vi "SUB_TextRunList_Color.vi"(3 "Current Step":i32, 4 "Totally Test Items":i32, 5 "List run file":string[](array[string])) -> (1 "ListFile":cluster{"Result":bool, string}[](array[cluster]))   [LabVIEW 2011]
panel:
  out "exeFilename":string
  in  "Result":bool
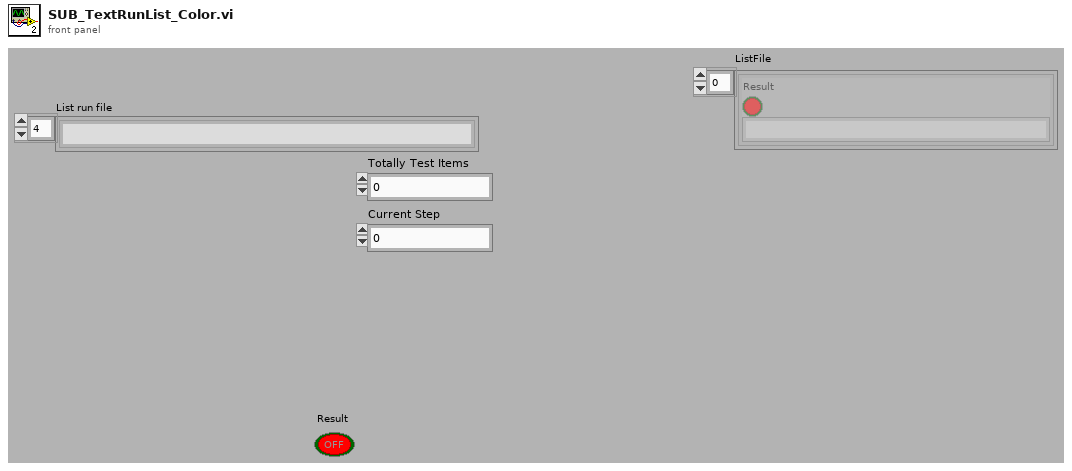
[diagram p1: front panel]
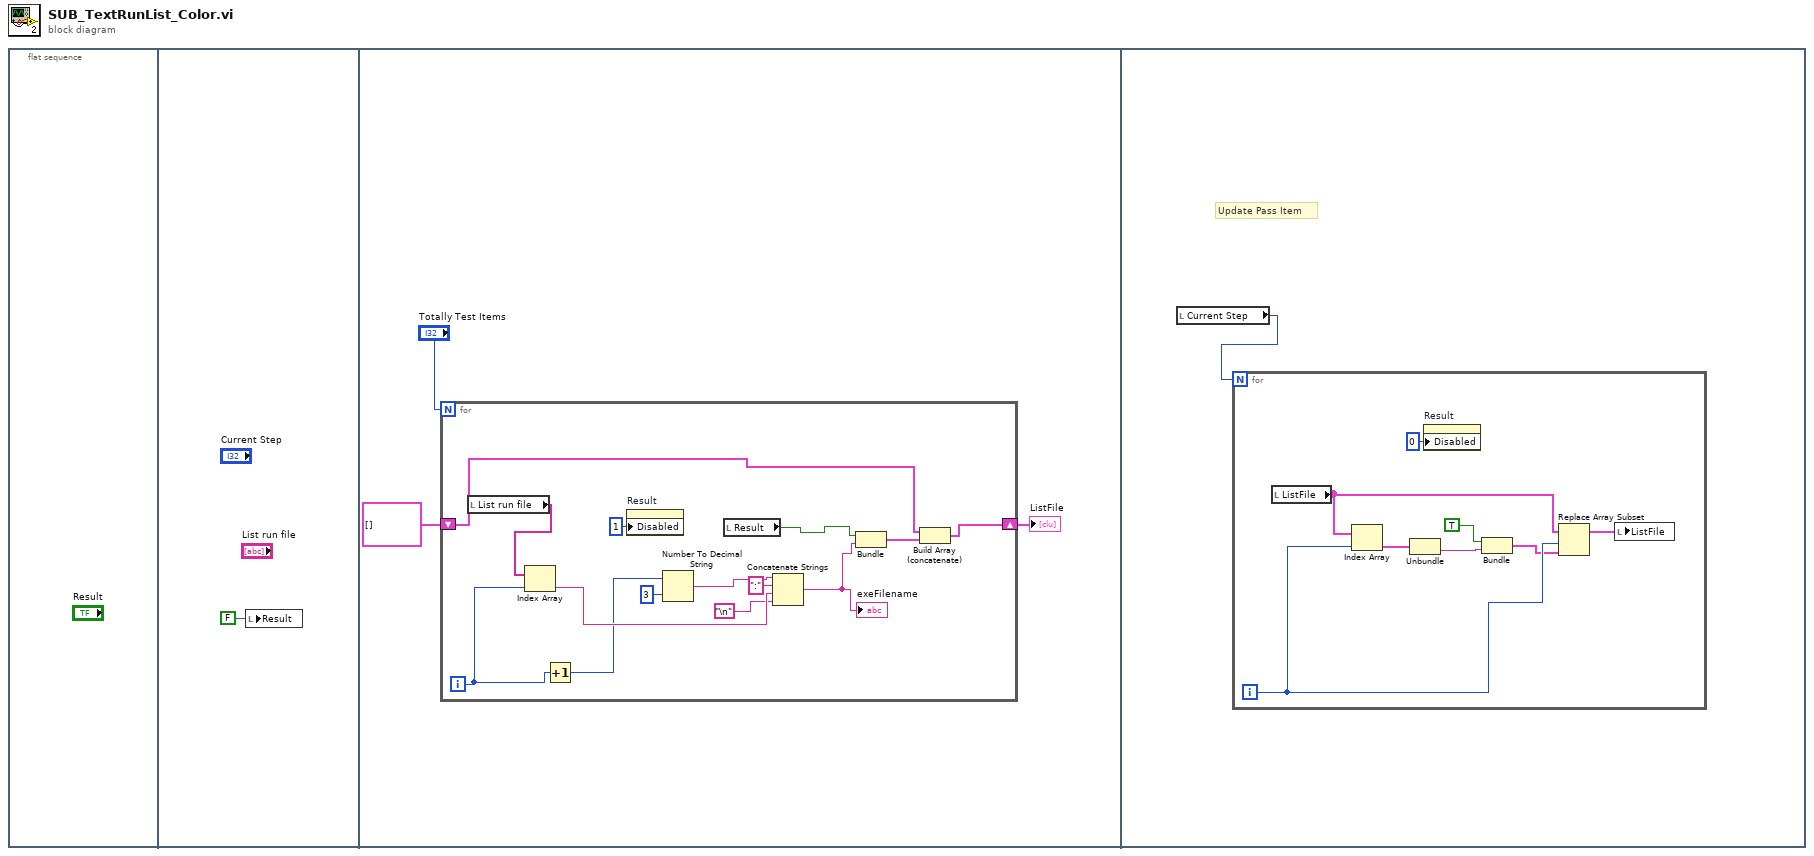
[diagram p0: block diagram]
diagram:
  n1 = flat-sequence {
    frame #0 {
    }
    frame #1 {
      n2 = local write "Result"(FALSE ("Result")) -> ()
    }
    frame #2 {
      n3 = for {
        N: "Totally Test Items" -> [_]
        shift-right: [w12] -> w3
        shift-left: cluster{"Result":bool, string}[] [] -> [w11]
        i -> [w8]
        n4 = local read "List run file"() -> (w18:string[])
        n5 = Index Array(array=w18, index=w8) -> (element=w14:string)
        n6 = Increment(x=w8) -> (x+1=w7:i32)
        n7 = property on="Result" class="Bool (strict)"("Disabled"=u8 1) -> ()  [unwired: 2 in, 2 out]
        n8 = Number To Decimal String(number=w7, width (-)=i16 3) -> (decimal integer string=w16:string)
        n9 = local read "Result"() -> (w6:bool)
        n10 = Concatenate Strings(w16, ":" ("string"), w14, "\n") -> (w10:string)
        "exeFilename" <- w10
        n11 = Bundle("Result"=w6, w10) -> (w9:cluster{"Result":bool, string})  [unwired: 1 in]
        n12 = Build Array (concatenate)(w11, w9) -> (w12:cluster{"Result":bool, string}[])
      }
      "ListFile" <- w3
    }
    frame #3 {
      # "Update Pass Item"
      n13 = local read "Current Step"() -> (w19:i32)
      n14 = for {
        N: w19 -> [_]
        i -> [w23]
        n15 = local read "ListFile"() -> (w24:cluster{"Result":bool, string}[])
        n16 = Index Array "Index Array"(array=w24, index=w23) -> (element=w27:cluster{"Result":bool, string})
        n17 = Unbundle(w27) -> (w26:string)  [unwired: 1 out]
        n18 = property on="Result" class="Bool (strict)"("Disabled"=u8 0) -> ()  [unwired: 2 in, 2 out]
        n19 = Bundle(TRUE, w26) -> (w22:cluster{bool, string})  [unwired: 1 in]
        n20 = Replace Array Subset "Replace Array Subset"(array=w24, new element=w22, index=w23) -> (w21:cluster{"Result":bool, string}[])
        n21 = local write "ListFile"(w21) -> ()
      }
    }
  }
